vi "testserialRT.vi"() -> ()   [LabVIEW 2017]
uses:
  <vilib>/Instr/_visa.llb/VISA Configure Serial Port (Instr).vi
panel:
  out "s? t:f":i32
  out "error out":errorcluster
  out "Decimal number 4":i32
  out "Decimal number 3":i32
  out "Decimal number 2":i32
  out "Decimal number":i32
  out "String":string
  in  "stop":bool
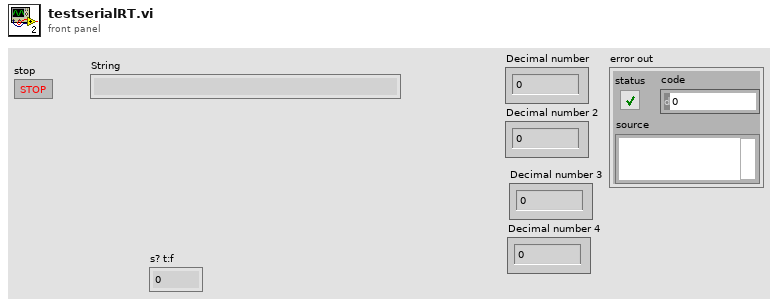
[diagram p1: front panel]
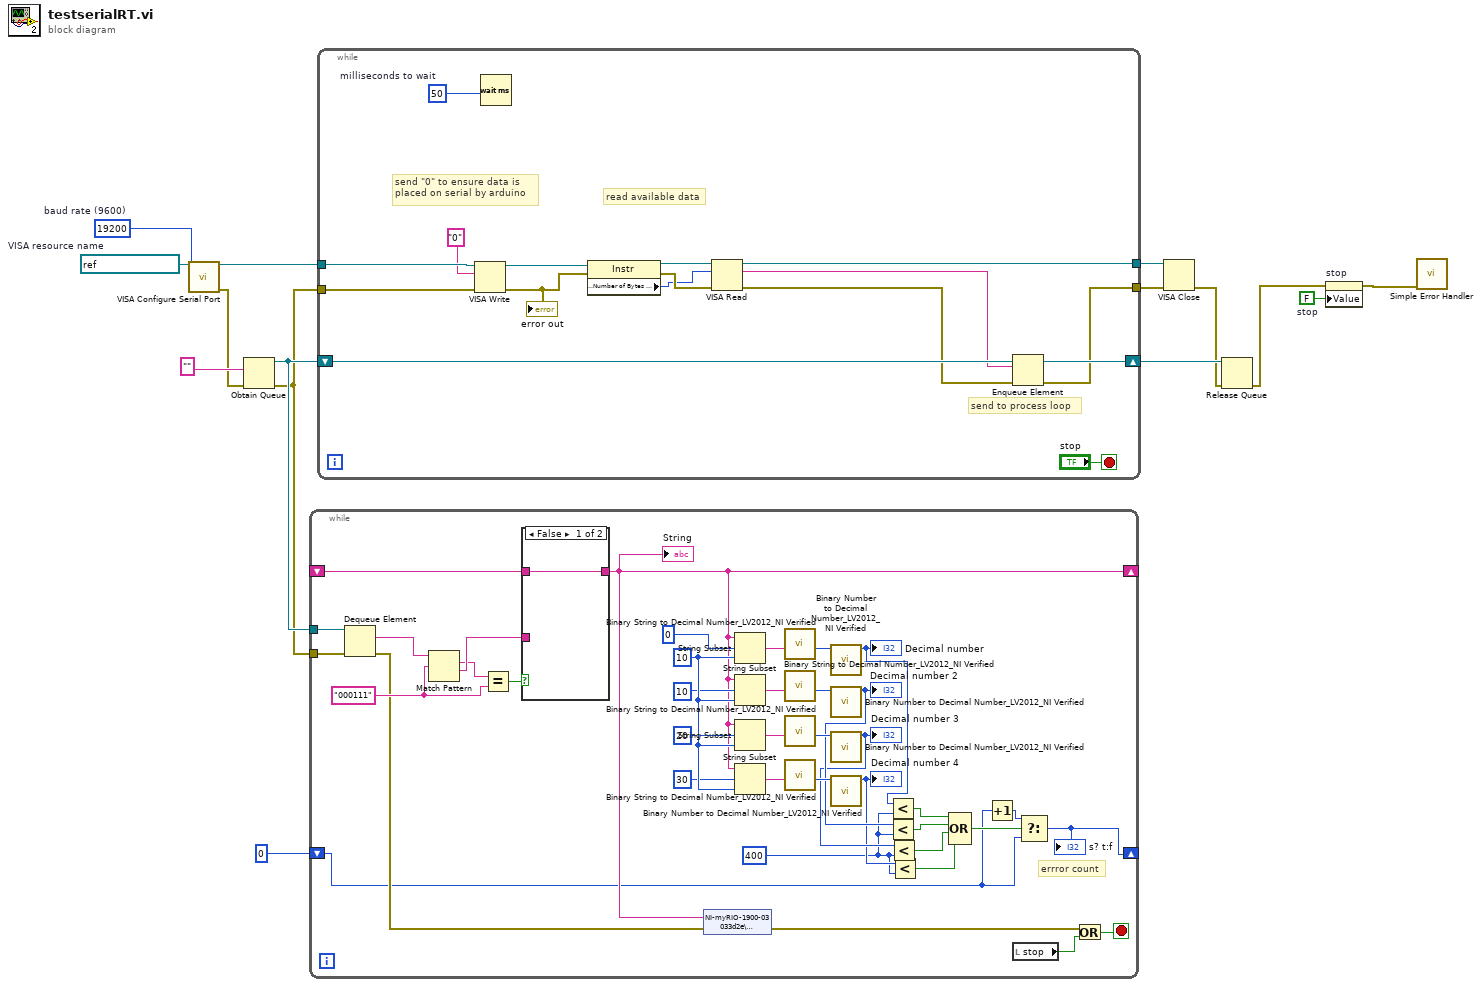
[diagram p0: block diagram]
diagram:
  w2 = u32 19200  # baud rate (9600)
  w3 = FALSE  # stop
  w15 = refnum<visa-resource-name> "ASRL2::INSTR"  # VISA resource name
  n1 = call-poly "VISA Configure Serial Port"("VISA resource name"=w15, "baud rate (9600)"=w2) -> ("VISA resource name out"=w14:refnum<visa-resource-name>, "error out"=w10:errorcluster)  [unwired: 12 in]
  n2 = Obtain Queue(element data type="", error in (no error)=w10) -> (queue out=w7:refnum<queue>, error out=w6:errorcluster)  [unwired: 3 in, 1 out]
  n3 = while {
    tunnel: w7 -> [w54]
    tunnel: w6 -> [w53]
    shift-right: [w29] -> _
    shift-left: _ -> [w45]
    shift-right: [w17] -> _
    shift-left: 0 -> [w18]
    stop <- w51 stop-if-true
    w16 = 400
    w36 = 10 ("length (rest)")
    w47 = "000111" ("y")
    # "errror count"
    n4 = Dequeue Element(queue=w54, error in (no error)=w53) -> (element=w49:string, error out=w31:errorcluster)  [unwired: 1 in, 2 out]
    n5 = Match Pattern(string=w49, regular expression=w47) -> (match substring=w46:string, after substring=w48:string)  [unwired: 1 in, 2 out]
    n6 = Equal?(x=w46, y=w47) -> (x = y?=w50:bool)
    n7 = case shown="False" w50 {
      tunnel: w48 -> [_ w56]
      tunnel: [w55 w56] -> w29
      tunnel: w45 -> [w55 _]
      frame False {
      }
      frame True {
      }
    }
    "String" <- w29
    n8 = shared-variable "NI-myRIO-1900-03033d2e\\sharedVariables.lvlib\\data"(w29, error in=w31) -> (error out=w30:errorcluster)
    n9 = String Subset(string=w29, offset (0)=0, length (rest)=w36) -> (substring=w37:string)
    n10 = String Subset(string=w29, offset (0)=10 ("length (rest)"), length (rest)=w36) -> (substring=w38:string)
    n11 = String Subset(string=w29, offset (0)=20 ("length (rest)"), length (rest)=w36) -> (substring=w39:string)
    n12 = String Subset(string=w29, offset (0)=30 ("length (rest)"), length (rest)=w36) -> (substring=w40:string)
    n13 = call "Binary String to Decimal Number_LV2012_NI Verified.vi"("String"=w37) -> ("Number"=w41:u64)  [unwired: 10 in]
    n14 = call "Binary String to Decimal Number_LV2012_NI Verified.vi"("String"=w38) -> ("Number"=w42:u64)  [unwired: 10 in]
    n15 = call "Binary String to Decimal Number_LV2012_NI Verified.vi"("String"=w39) -> ("Number"=w43:u64)  [unwired: 10 in]
    n16 = call "Binary String to Decimal Number_LV2012_NI Verified.vi"("String"=w40) -> ("Number"=w44:u64)  [unwired: 10 in]
    n17 = call "Binary Number to Decimal Number_LV2012_NI Verified.vi"("Binary number"=w41) -> ("Decimal number"=w28:i32)  [unwired: 10 in]
    "Decimal number" <- w28
    n18 = call "Binary Number to Decimal Number_LV2012_NI Verified.vi"("Binary number"=w42) -> ("Decimal number"=w26:i32)  [unwired: 10 in]
    "Decimal number 2" <- w26
    n19 = call "Binary Number to Decimal Number_LV2012_NI Verified.vi"("Binary number"=w43) -> ("Decimal number"=w24:i32)  [unwired: 10 in]
    "Decimal number 3" <- w24
    n20 = call "Binary Number to Decimal Number_LV2012_NI Verified.vi"("Binary number"=w44) -> ("Decimal number"=w22:i32)  [unwired: 10 in]
    "Decimal number 4" <- w22
    n21 = Less?(x=w28, y=w16) -> (x < y?=w27:bool)
    n22 = Less?(x=w26, y=w16) -> (x < y?=w25:bool)
    n23 = Less?(x=w24, y=w16) -> (x < y?=w23:bool)
    n24 = Less?(x=w22, y=w16) -> (x < y?=w21:bool)
    n25 = Compound Arithmetic op=OR(w27, w25, w23, w21) -> (w20:bool)
    n26 = Increment(x=w18) -> (x+1=w19:i32)
    n27 = local read "stop"() -> (w52:bool)
    n28 = Select(t=w19, s=w20, f=w18) -> (s? t:f=w17:i32)
    "s? t:f" <- w17
    n29 = Or(x=w30, y=w52) -> (x .or. y?=w51:bool)
  }
  n30 = while {
    tunnel: w14 -> [w71]
    tunnel: w6 -> [w70]
    tunnel: [w58] -> w13
    tunnel: [w66] -> w12
    shift-right: [w69] -> w9
    shift-left: w7 -> [w67]
    stop <- "stop" stop-if-true
    w68 = u32 50  # milliseconds to wait
    # "send to process loop"
    # "read available data"
    # "send \"0\" to ensure data is\nplaced on serial by arduino"
    n31 = VISA Write(VISA resource name=w71, write buffer="0", error in (no error)=w70) -> (VISA resource name out=w60:refnum<visa-resource-name>, error out=w59:errorcluster)  [unwired: 1 out]
    "error out" <- w59
    n32 = Wait (ms)(milliseconds to wait=w68) -> ()  [unwired: 1 out]
    n33 = property class="Instr"(reference=w60, error in=w59) -> (reference out=w64:refnum<visa-resource-name>, error out=w63:errorcluster, "Serial Settings:Number of Bytes at Serial Port"=w62:u32)
    n34 = VISA Read(VISA resource name=w64, byte count=w62, error in (no error)=w63) -> (VISA resource name out=w58:refnum<visa-resource-name>, read buffer=w65:string, error out=w57:errorcluster)  [unwired: 1 out]
    n35 = Enqueue Element(queue=w67, element=w65, error in (no error)=w57) -> (queue out=w69:refnum<queue>, error out=w66:errorcluster)  [unwired: 1 in, 1 out]
  }
  n36 = VISA Close(VISA resource name=w13, error in (no error)=w12) -> (error out=w8:errorcluster)
  n37 = Release Queue(queue=w9, error in (no error)=w8) -> (error out=w5:errorcluster)  [unwired: 1 in, 2 out]
  n38 = property on="stop" class="Bool (strict)"(error in=w5, "Value"=w3) -> (error out=w4:errorcluster)  [unwired: 1 in, 1 out]
  n39 = call <vilib>:"Simple Error Handler.vi"("error in (no error)"=w4) -> ()  [unwired: 4 in, 5 out]
